vi "Write Measurement Variance.vi"(8 "error in (no error)":errorcluster, 10 "Measurement Variance":dbl, 11 "Kalman_Filter in":refnum<class "Kalman_Filter.lvclass">) -> (0 "error out":errorcluster, 3 "Kalman_Filter out":refnum<class "Kalman_Filter.lvclass">)   [LabVIEW 2021, in "Kalman_Filter.lvclass"]
uses:
  Kalman_Filter.lvclass
  Kalman_Filter.lvclass/Kalman_Filter.ctl
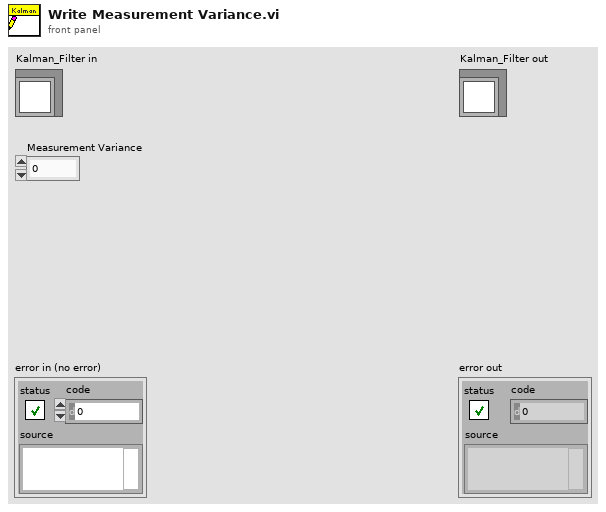
[diagram p1: front panel]
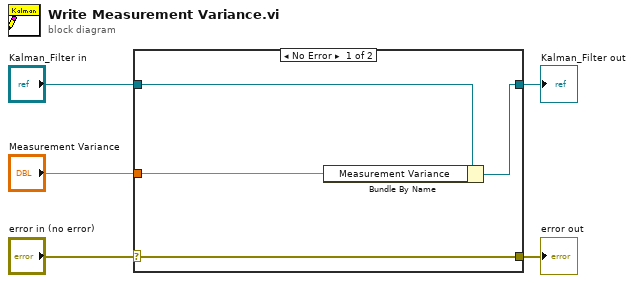
[diagram p0: block diagram]
diagram:
  n1 = case shown="No Error" "error in (no error)" {
    selector: "error in (no error)" -> [w9 w10]
    tunnel: [w9 w10] -> w4
    tunnel: [w7 w11] -> w2
    tunnel: "Kalman_Filter in" -> [w8 w11]
    tunnel: "Measurement Variance" -> [w6 _]
    frame No Error {
      n2 = Bundle By Name(cluster=w8, "Measurement Variance"=w6) -> (w7:refnum<class "Kalman_Filter.lvclass">)
    }
    frame Error {
    }
  }
  "error out" <- w4
  "Kalman_Filter out" <- w2
